vi "Simulation.vi"() -> ()   [LabVIEW 2023]
panel:
  out "Picture":picture
  out "Field":cluster{cluster{dbl, dbl}[]}[](graph)
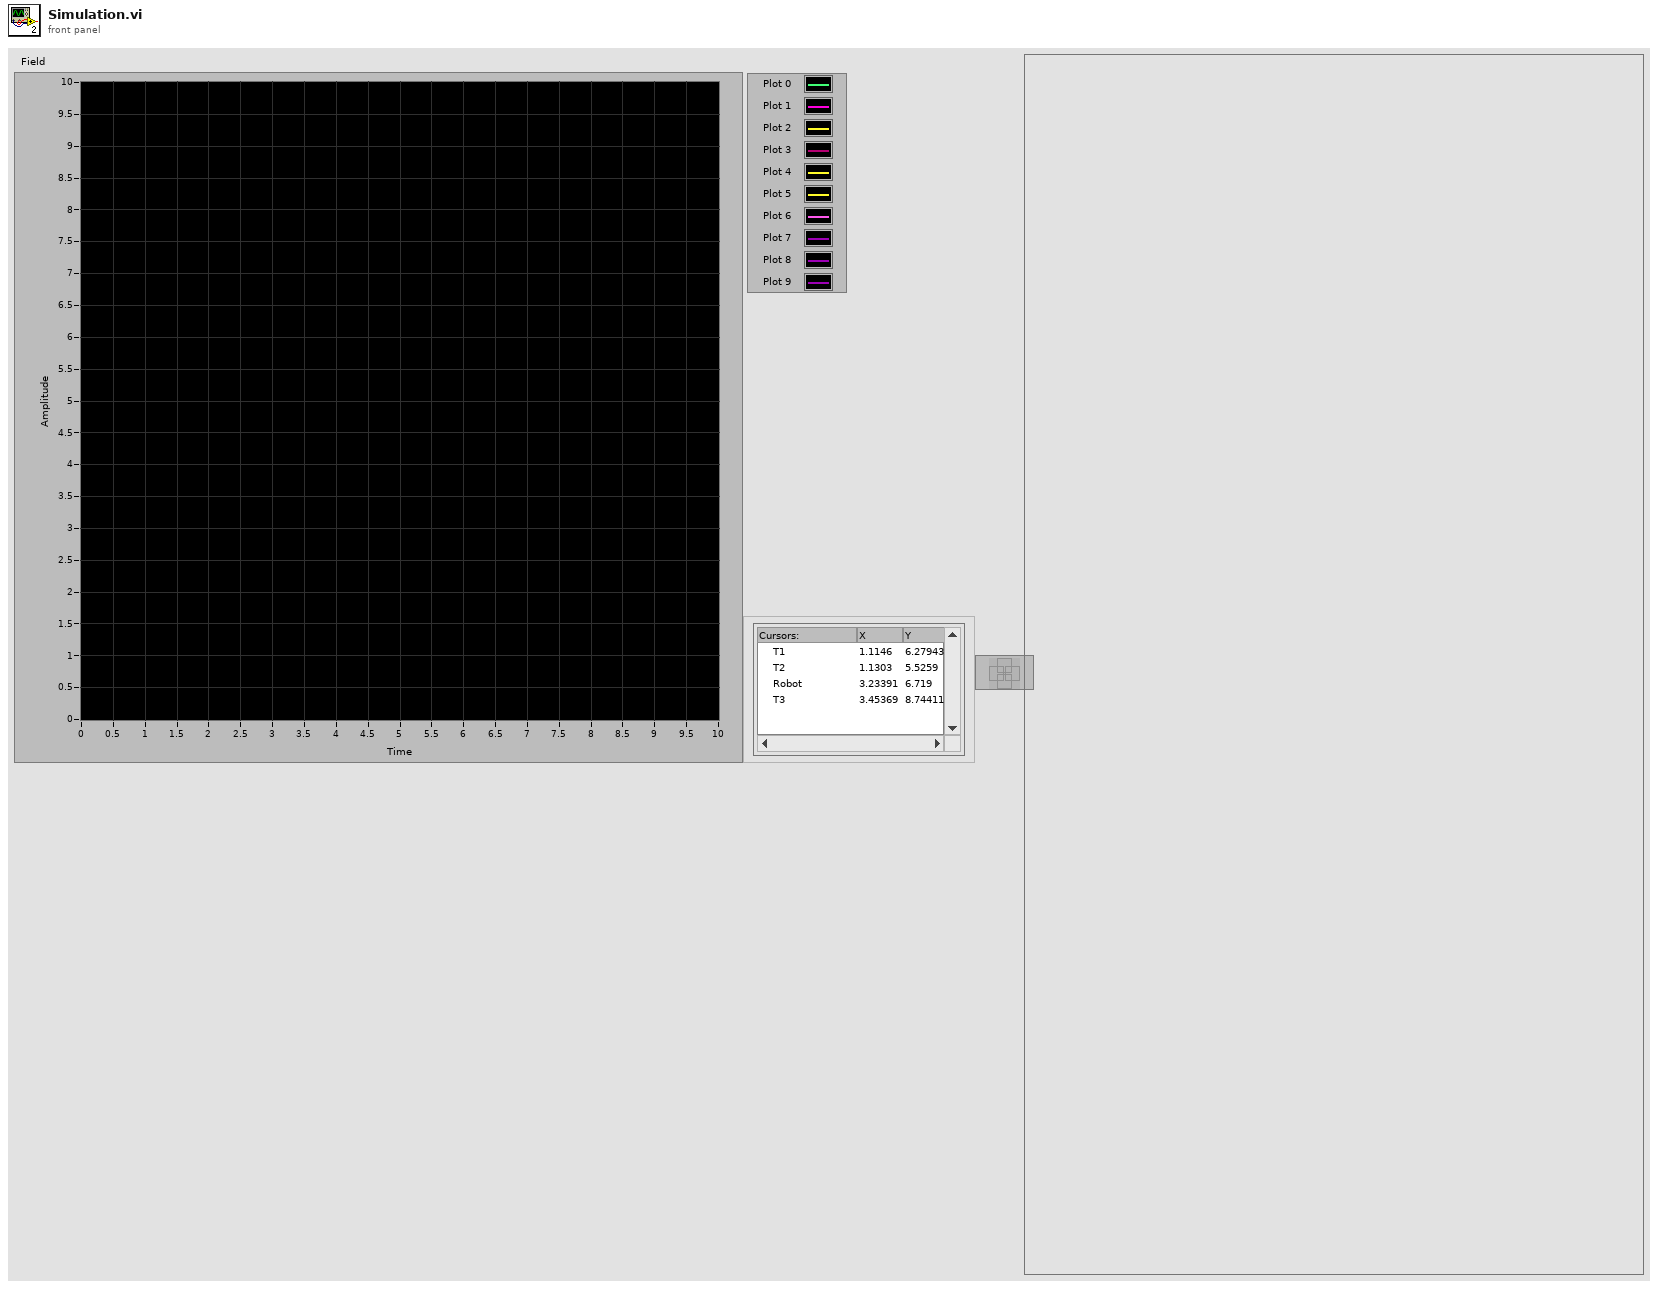
[diagram p1: front panel]
types:
  T1 = typedef "LVCursorListTypeDef.ctl" = cluster{"Name":string, "Color":u32, "Style":u8, "Point Style":u8, "Name Visible":bool, "Allow Drag":bool, "Cursor Mode":u32, "Plot":i32, "Index":i32, "Position":cluster{"X":dbl, "Y":dbl}, "X Scale":u32, "Y Scale":u32, "Watch Plots":i32[], "Watch All Plots":bool, "Plot Area":i32, "Label Offset":cluster{"X":dbl, "Y":dbl}}[]
  T2 = cluster{"Name":string, "Color":u32, "Style":u8, "Point Style":u8, "Name Visible":bool, "Allow Drag":bool, "Cursor Mode":u32, "Plot":i32, "Index":i32, "Position":cluster{"X":dbl, "Y":dbl}, "X Scale":u32, "Y Scale":u32, "Watch Plots":i32[], "Watch All Plots":bool, "Plot Area":i32, "Label Offset":cluster{"X":dbl, "Y":dbl}}
  T3 = cluster{"angle - deg":dbl, "Position":cluster{"X":dbl, "Y":dbl}}
  T4 = cluster{"cluster":cluster{"angle - deg":dbl, "Position":cluster{"X":dbl, "Y":dbl}}, "cluster":cluster{"angle - deg":dbl, "Position":cluster{"X":dbl, "Y":dbl}}}
  T5 = cluster{i32, "Pt Test Results":enum16{"Miss", "Rect Hit", "Arrow Hit"}}
  T6 = cluster{"center":cluster{"X":sgl, "Y":sgl}, "radius":sgl}
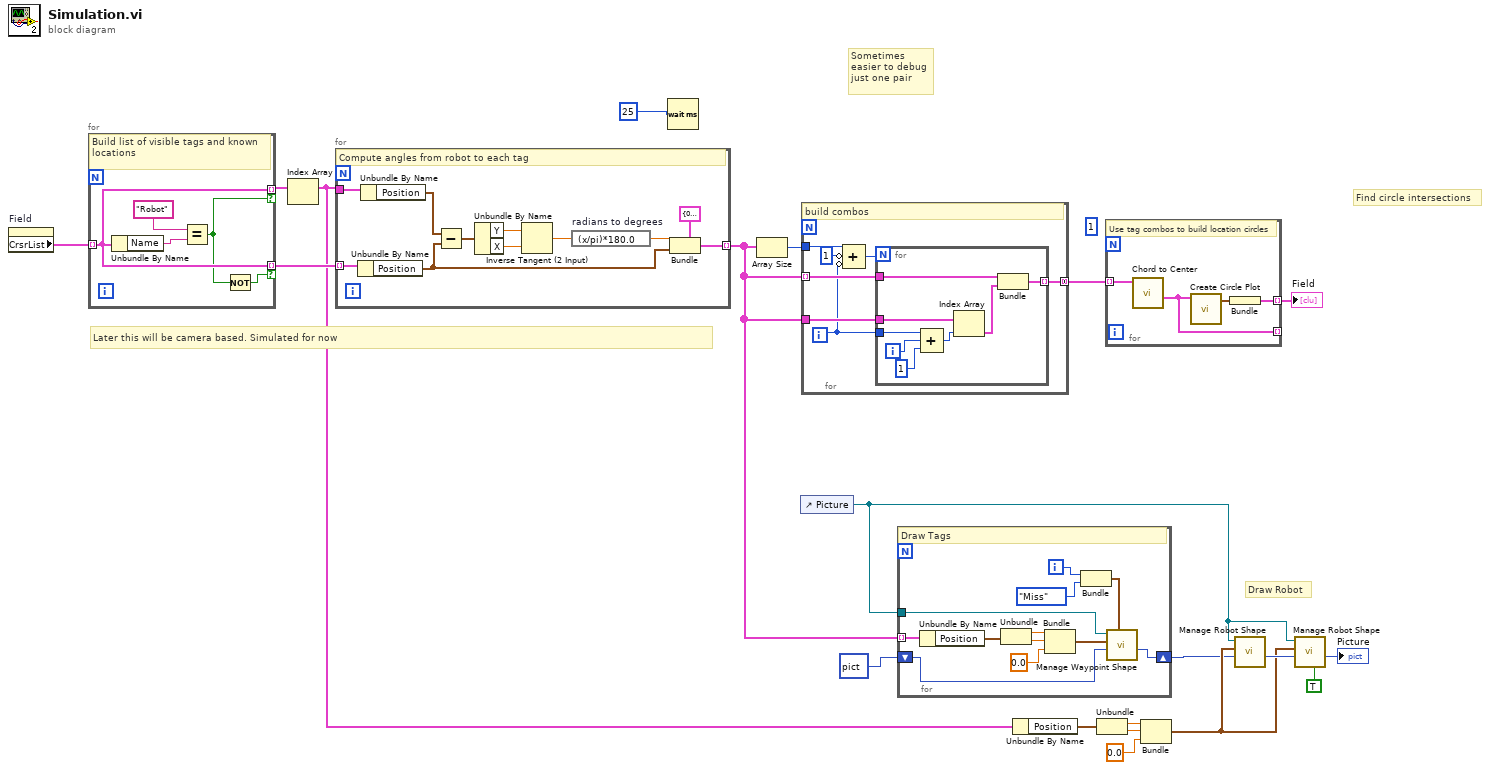
[diagram p0: block diagram]
diagram:
  (unwired) u32 1 ("milliseconds to wait")
  # "Draw Robot"
  # "Find circle intersections"
  # "Sometimes\neasier to debug\njust one pair"
  # "Later this will be camera based. Simulated for now"
  n1 = property on="Field" class="XYGraph (strict)"() -> ("CrsrList"=w20:T1)  [unwired: 2 in, 2 out]
  n2 = for {
    tunnel: w20 -> [w23] mode=indexing
    tunnel: [w23] -> w19 mode=indexing if=w22
    tunnel: [w23] -> w18 mode=indexing if=w21
    # "Build list of visible tags and known locations"
    n3 = Unbundle By Name(w23) -> ("Name"=w25:string)
    n4 = Equal?(x="Robot", y=w25) -> (x = y?=w22:bool)
    n5 = Not(x=w22) -> (.not. x?=w21:bool)
  }
  n6 = Index Array(array=w19) -> (element=w11:T2)  [unwired: 1 in]
  n7 = for {
    tunnel: w11 -> [w36]
    tunnel: w18 -> [w35] mode=indexing
    tunnel: [w28] -> w12 mode=indexing
    # "Compute angles from robot to each tag"
    n8 = Unbundle By Name(w35) -> ("Position"=w29:cluster{"X":dbl, "Y":dbl})
    n9 = Unbundle By Name(w36) -> ("Position"=w34:cluster{"X":dbl, "Y":dbl})
    n10 = Subtract(x=w34, y=w29) -> (x-y=w33:cluster{"X":dbl, "Y":dbl})
    n11 = Unbundle By Name(w33) -> ("Y"=w32:dbl, "X"=w31:dbl)
    n12 = Inverse Tangent (2 Input)(1:w31, 2:w32) -> (0:w30:dbl)
    n13 = expression code="(x/pi)*180.0" "radians to degrees"(w30) -> (w27:dbl)
    n14 = Bundle(cluster=T3 {"angle - deg"=0.0, "Position"={"X"=0.0, "Y"=0.0}}, "angle - deg"=w27, "Position"=w29) -> (w28:T3)
  }
  n15 = Wait (ms)(milliseconds to wait=u32 25) -> ()  [unwired: 1 out]
  n16 = Array Size(array=w12) -> (size(s)=w16:i32)
  n17 = control-ref of="Picture"() -> (w1:refnum<vi>)
  n18 = for {
    tunnel: w12 -> [w43] mode=indexing
    tunnel: w12 -> [w42]
    tunnel: [w41] -> w15 mode=concatenating
    tunnel: w16 -> [w39]
    i -> [w38]
    # "build combos"
    n19 = Compound Arithmetic op=ADD(w39, invert 1 ("value"), invert w38) -> (w40:i32)
    n20 = for {
      N: w40 -> [_]
      tunnel: w43 -> [w51]
      tunnel: w42 -> [w50]
      tunnel: w38 -> [w47]
      tunnel: [w44] -> w41 mode=indexing
      i -> [w46]
      n21 = Compound Arithmetic op=ADD(w47, w46, 1 ("value")) -> (w48:i32)
      n22 = Index Array(array=w50, index=w48) -> (element=w49:T3)
      n23 = Bundle("cluster"=w51, "cluster"=w49) -> (w44:T4)  [unwired: 1 in]
    }
  }
  n24 = for {
    tunnel: w1 -> [w63]
    shift-right: [w52] -> w2
    shift-left: picture data[5B] ("new picture out") -> [w62]
    tunnel: w12 -> [w61] mode=indexing
    i -> [w55]
    # "Draw Tags"
    n25 = Unbundle By Name(w61) -> ("Position"=w59:cluster{"X":dbl, "Y":dbl})
    n26 = Unbundle(w59) -> ("X"=w60:dbl, "Y"=w58:dbl)
    n27 = Bundle("X"=w60, "Y"=w58, "th"=0.0) -> (w56:cluster{"X":dbl, "Y":dbl, "th":dbl})  [unwired: 1 in]
    n28 = Bundle(w55, "Pt Test Results"=enum16{"Miss", "Rect Hit", "Arrow Hit"}."Miss") -> (w53:T5)  [unwired: 1 in]
    n29 = call "Manage Waypoint Shape.vi"("Drawing Options"=w53, "new picture in"=w62, "Waypoint Position (ft)"=w56, "Pict Ref"=w63) -> ("new picture out"=w52:picture)  [unwired: 6 in, 1 out]
  }
  n30 = Unbundle By Name(w11) -> ("Position"=w8:cluster{"X":dbl, "Y":dbl})
  n31 = Unbundle(w8) -> ("X"=w7:dbl, "Y"=w9:dbl)
  n32 = for {
    tunnel: w15 -> [w65] mode=indexing
    tunnel: [w66] -> w14 mode=indexing
    tunnel: [w64] -> _ mode=indexing
    # "Use tag combos to build location circles"
    n33 = call "Chord to Center.vi"("Tag points"=w65) -> ("output circle info"=w64:T6)  [unwired: 7 in, 3 out]
    n34 = call "Create Circle Plot.vi"("Circle Descr"=w64) -> ("Points"=w67:cluster{dbl, dbl}[])  [unwired: 10 in]
    n35 = Bundle("Points"=w67) -> (w66:cluster{"Points":cluster{dbl, dbl}[]})  [unwired: 1 in]
  }
  "Field" <- w14
  n36 = Bundle("X"=w7, "Y"=w9, "th"=0.0) -> (w4:cluster{"X":dbl, "Y":dbl, "th":dbl})  [unwired: 1 in]
  n37 = call "Manage Robot Shape.vi"("new picture in"=w2, "Robot Position (ft)"=w4, "Pict Ref"=w1) -> ("new picture out"=w6:picture)  [unwired: 6 in, 2 out]
  n38 = call "Manage Robot Shape.vi"("Lighter"=TRUE ("Outline"), "new picture in"=w6, "Robot Position (ft)"=w4, "Pict Ref"=w1) -> ("new picture out"=→"Picture":picture)  [unwired: 5 in, 2 out]
